vi "ReadSGL.vi"(11 "Address":u32) -> (3 "Data":sgl)   [LabVIEW 2016]
uses:
  <vilib>/rvi/Memory/Memory_Emulation/nirvimemoryFastEmulation.vi
  <vilib>/rvi/Memory/Memory_Emulation/nirvimemoryEmulation.vi
  <vilib>/rvi/Emulation/niFpgaEmulationIsFPGAContextNoSignature.vi
  <vilib>/rvi/DataTransferAndStorage/Container/Common/niFpgaContainerGetUniqueNameForEmu.vi
  <vilib>/rvi/Emulation/niFpgaProcessEmulError.vi
  <vilib>/rvi/Emulation/niFpgaSctlEmulationGetInTimedLoop.vi
  <vilib>/rvi/errors/nirviReportUnexpectedCaseInternalError (U32).vi
  <vilib>/rvi/DataTransferAndStorage/Container/Common/niFpgaContainerExecOnDevCompGetState.vi
  <vilib>/rvi/Memory/Memory_Emulation/niFpgaMemoryEmulationCacheClearOnFirstRun.vi
  <vilib>/rvi/Memory/Memory_Emulation/nirvimemoryEmulationManagerCache_MakeExclusive.vi
  <vilib>/rvi/Memory/Memory_Emulation/niFpgaMemoryEmulationValidateCache.vi
  <vilib>/rvi/Memory/Memory_Emulation/nirvimemoryEmulationManagerCache_InsertValue.vi
  <vilib>/Utility/error.llb/Clear Errors.vi
  <vilib>/rvi/Memory/Memory_Emulation/nirvimemoryEmulationManagerCache_ReleaseExclusive.vi
  <vilib>/rvi/Memory/Memory_Emulation/nirvimemoryEmulationManagerCache_GetValue.vi
  <vilib>/rvi/Memory/Memory_Emulation/nirvimemoryEmulationManagerCache_SetValue.vi
  <vilib>/rvi/Emulation/niFpgaSctlEmulationResourceMgr.vi
  <vilib>/rvi/DataTransferAndStorage/Container/XNode/niFpgaContainer.xnode
  <vilib>/rvi/Memory/Memory_Emulation/niFpgaMemoryEmulationRefIn.vi
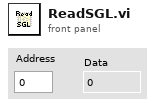
[diagram p1: front panel]
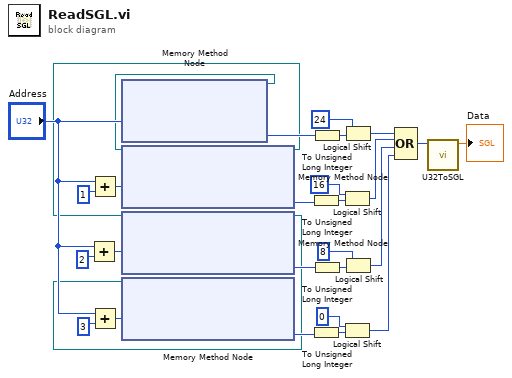
[diagram p0: block diagram]
diagram:
  n1 = Add(x="Address", y=u32 2) -> (x+y=w10:u32)
  n2 = Add(x="Address", y=u32 1) -> (x+y=w20:u32)
  n3 = Add(x="Address", y=u32 3) -> (x+y=w19:u32)
  n4 = xnode ("Memory Method Node")("Address"="Address") -> ("Data"=w28:u8, "Memory Out"=w5:refnum<k21>)  [unwired: 1 in]
  n5 = xnode ("Memory Method Node")("Address"=w20, "Memory In"=w5) -> ("Data"=w24:u8, "Memory Out"=w4:refnum<k21>)
  n6 = xnode ("Memory Method Node")("Address"=w10, "Memory In"=w4) -> ("Data"=w12:u8, "Memory Out"=w3:refnum<k21>)
  n7 = xnode ("Memory Method Node")("Address"=w19, "Memory In"=w3) -> ("Data"=w16:u8)  [unwired: 1 out]
  n8 = To Unsigned Long Integer(number=w24) -> (unsigned 32bit integer=w25:u32)
  n9 = To Unsigned Long Integer(number=w16) -> (unsigned 32bit integer=w15:u32)
  n10 = To Unsigned Long Integer(number=w28) -> (unsigned 32bit integer=w27:u32)
  n11 = To Unsigned Long Integer(number=w12) -> (unsigned 32bit integer=w13:u32)
  n12 = Logical Shift(y=i16 16, x=w25) -> (x << y=w22:u32)
  n13 = Logical Shift(y=i16 0, x=w15) -> (x << y=w7:u32)
  n14 = Logical Shift(y=i16 24, x=w27) -> (x << y=w6:u32)
  n15 = Logical Shift(y=i16 8, x=w13) -> (x << y=w8:u32)
  n16 = Compound Arithmetic op=OR(w6, w22, w8, w7) -> (w2:u32)
  n17 = call "U32ToSGL.vi"("U32"=w2) -> ("SGL"=→"Data":sgl)  [unwired: 10 in]
